vi "2021_day6_task2_sub.vi"(9 "Numeric in":i32, 10 "Array in":i8[](array[numeric]), 11 "# of Iteration":i32) -> (1 "Array len":i32, 2 "Array out":i8[](array[numeric]), 4 "Arr to overflow":i32, 6 "Iteration":i32)   [LabVIEW 2021]
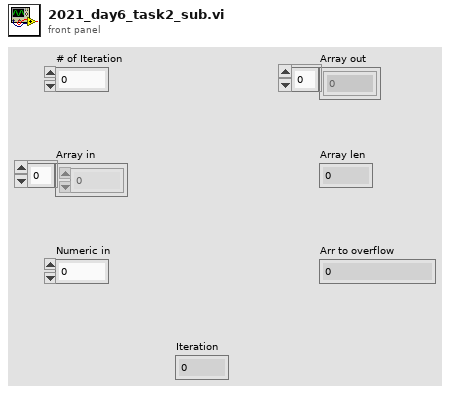
[diagram p1: front panel]
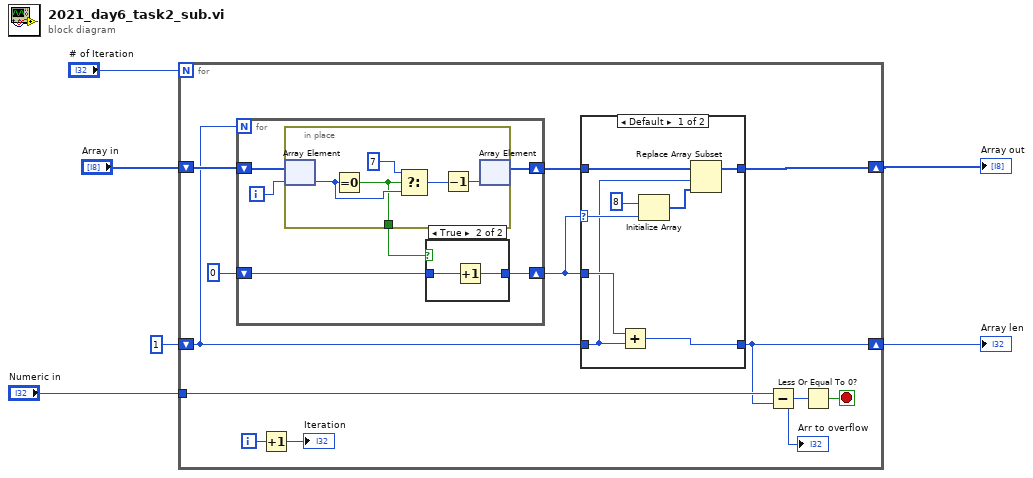
[diagram p0: block diagram]
diagram:
  n1 = for {
    N: "# of Iteration" -> [_]
    shift-right: [w12] -> w6
    shift-left: "Array in" -> [w14]
    shift-right: [w10] -> w4
    shift-left: 1 -> [w9]
    tunnel: "Numeric in" -> [w16]
    i -> [w17]
    stop <- w15 stop-if-true
    n2 = for {
      N: w9 -> [_]
      shift-right: [w32] -> w18
      shift-left: w14 -> [w34]
      shift-right: [w30] -> w11
      shift-left: 0 -> [w31]
      i -> [w33]
      n3 = in-place {
        in-place-border: [w39] -> w29
        n4 = in-place-array #1(w34, w33) -> (w40:i8)
        n5 = Equal To 0?(x=w40) -> (x = 0?=w39:bool)
        n6 = Select(t=i8 7, s=w39, f=w40) -> (s? t:f=w41:i8)
        n7 = Decrement(x=w41) -> (x-1=w38:i8)
        n8 = in-place-array #1(w38) -> (w32:i8[])  [unwired: 1 out]
      }
      n9 = case shown="True" w29 {
        tunnel: w31 -> [w35 w37]
        tunnel: [w35 w36] -> w30
        frame False {
        }
        frame True {
          n10 = Increment(x=w37) -> (x+1=w36:i32)
        }
      }
    }
    n11 = Increment(x=w17) -> (x+1=→"Iteration":i32)
    n12 = case shown="Default" w11 {
      selector: w11 -> [w23 _]
      tunnel: w18 -> [w26 w28]
      tunnel: [w25 w28] -> w12
      tunnel: w11 -> [w21 _]
      tunnel: w9 -> [w19 w27]
      tunnel: [w20 w27] -> w10
      frame Default {
        n13 = Add(x=w21, y=w19) -> (x+y=w20:i32)
        n14 = Initialize Array(i8 8, w23) -> (w24:i8[])
        n15 = Replace Array Subset(array=w26, new element=w24, index=w19) -> (w25:i8[])
      }
      frame 0 {
      }
    }
    n16 = Subtract(x=w16, y=w10) -> (x-y=w8:i32)
    "Arr to overflow" <- w8
    n17 = Less Or Equal To 0?(x=w8) -> (x <= 0?=w15:bool)
  }
  "Array out" <- w6
  "Array len" <- w4
